vi "SendBodeData.vi"(7 "STM Message String":string="RT: GetBodeData", 8 "error in (no error)":errorcluster, 9 "Phase Array":cluster{"Freq":dbl[], "Phase":dbl[]}, 10 "Magnitude Array":cluster{"Freq":dbl[], "Mag":dbl[]}, 11 "connection info in":T1) -> (0 "error out":errorcluster, 3 "connection info out":T1)   [LabVIEW 2020, in "DynamicSignalAnalyzer.lvlib"]
doc: "Unwrap phase and send bode data via STM from RT target to Host PC"
uses:
  DynamicSignalAnalyzer.lvlib
  <vilib>/NI/STM/TCP/TCP Connection Info.ctl
  <vilib>/NI/STM/SubVIs/MetaDataElement.ctl
  TypeDefs/BodePlot.ctl
  <vilib>/NI/STM/TCP/Write Message (TCP).vi
  <vilib>/Analysis/NI_AALPro.lvlib
  <vilib>/NI/STM/NI STM.lvlib
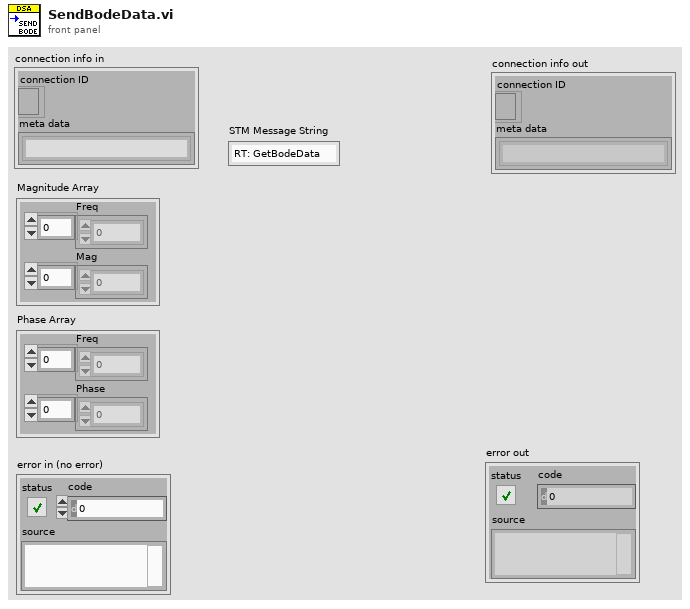
[diagram p1: front panel]
types:
  T1 = typedef "NI STM.lvlib/TCP Connection Info.ctl" = cluster{"connection ID":refnum<k5>, "meta data":T2[]}
  T2 = typedef "NI STM.lvlib/MetaDataElement.ctl" = string
  T3 = typedef "DynamicSignalAnalyzer.lvlib/BodePlot.ctl" = cluster{"Frequency [Hz]":dbl[], "Magnitude [abs]":dbl[], "Phase [deg]":dbl[]}
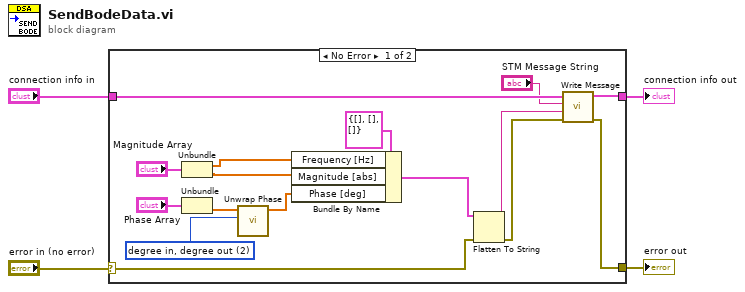
[diagram p0: block diagram]
diagram:
  n1 = case shown="No Error" "error in (no error)" {
    selector: "error in (no error)" -> [w11 w22]
    tunnel: [w6 w22] -> w3
    tunnel: "connection info in" -> [w9 w21]
    tunnel: [w8 w21] -> w1
    frame No Error {
      w17 = 2 items=["radian in, radian out", "radian in, degree out", "degree in, degree out", "degree in, radian out"] ("phase unit")
      n2 = Unbundle("Magnitude Array") -> ("Freq"=w15:dbl[], "Mag"=w5:dbl[])
      n3 = Unbundle("Phase Array") -> ("Phase"=w18:dbl[])  [unwired: 1 out]
      n4 = call <vilib>:"Unwrap Phase.vi"("phase unit"=w17, "Phase"=w18) -> ("Unwrapped Phase"=w14:dbl[])  [unwired: 8 in, 1 out]
      n5 = Bundle By Name(cluster=T3 {"Frequency [Hz]"=[], "Magnitude [abs]"=[], "Phase [deg]"=[]} ("Bode Plots"), "Frequency [Hz]"=w15, "Magnitude [abs]"=w5, "Phase [deg]"=w14) -> (w12:T3)
      n6 = Flatten To String(anything=w12, error in (no error)=w11) -> (data string=w13:string, error out=w10:errorcluster)  [unwired: 2 in, 1 out]
      n7 = call-poly <vilib>:"Write Message.vi"("error in"=w10, "data"=w13, "name"="STM Message String", "connection info in"=w9) -> ("error out"=w6:errorcluster, "connection info out"=w8:T1)  [unwired: 6 in]
    }
    frame Error {
    }
  }
  "connection info out" <- w1
  "error out" <- w3
